vi "ImageThreshold.vi"(2 "Noise standard deviation":dbl format="%.2f", 4 "Sky Scan":dbl[][](graph)=[[180.0, 184.0, 210.0, 205.0, 212.0, 190.0, 183.0, 167.0, 174.0, 172.0, 167.0], [160.0, 192.0, 193.0, 215.0, 200.0, 218.0, 195.0, 180.0, 189.0, 182.0, 179.0], [178.0, 191.0, 222.0, 308.0, 243.0, 199.0, 189.0, 200.0, 192.0, 188.0, 190.0], [170.0, 237.0, 250.0, 257.0, 352.0, 202.0, 187.0, 190.0, 176.0, 182.0, 185.0], [169.0, 264.0, 386.0, 656.0, 212.0, 209.0, 194.0, 190.0, 159.0, 169.0, 190.0], [176.0, 268.0, 1507.0, 3786.0, 748.0, 194.0, 190.0, 209.0, 181.0, 181.0, 174.0], [185.0, 271.0, 1969.0, 5368.0, 1397.0, 218.0, 210.0, 173.0, 194.0, 182.0, 194.0], [185.0, 236.0, 1172.0, 3209.0, 836.0, 187.0, 207.0, 185.0, 179.0, 191.0, 192.0], [169.0, 235.0, 428.0, 829.0, 280.0, 204.0, 175.0, 179.0, 169.0, 195.0, 199.0], [181.0, 195.0, 248.0, 349.0, 318.0, 185.0, 187.0, 188.0, 183.0, 184.0, 197.0], [170.0, 181.0, 186.0, 230.0, 225.0, 199.0, 191.0, 174.0, 181.0, 178.0, 184.0]]) -> (0 "Something ?":bool, 1 "Sky map threshold":dbl[][](graph)=[[180.0, 184.0, 210.0, 205.0, 212.0, 190.0, 183.0, 167.0, 174.0, 172.0, 167.0], [160.0, 192.0, 193.0, 215.0, 200.0, 218.0, 195.0, 180.0, 189.0, 182.0, 179.0], [178.0, 191.0, 222.0, 308.0, 243.0, 199.0, 189.0, 200.0, 192.0, 188.0, 190.0], [170.0, 237.0, 250.0, 257.0, 352.0, 202.0, 187.0, 190.0, 176.0, 182.0, 185.0], [169.0, 264.0, 386.0, 656.0, 212.0, 209.0, 194.0, 190.0, 159.0, 169.0, 190.0], [176.0, 268.0, 1507.0, 3786.0, 748.0, 194.0, 190.0, 209.0, 181.0, 181.0, 174.0], [185.0, 271.0, 1969.0, 5368.0, 1397.0, 218.0, 210.0, 173.0, 194.0, 182.0, 194.0], [185.0, 236.0, 1172.0, 3209.0, 836.0, 187.0, 207.0, 185.0, 179.0, 191.0, 192.0], [169.0, 235.0, 428.0, 829.0, 280.0, 204.0, 175.0, 179.0, 169.0, 195.0, 199.0], [181.0, 195.0, 248.0, 349.0, 318.0, 185.0, 187.0, 188.0, 183.0, 184.0, 197.0], [170.0, 181.0, 186.0, 230.0, 225.0, 199.0, 191.0, 174.0, 181.0, 178.0, 184.0]])   [LabVIEW 2009]
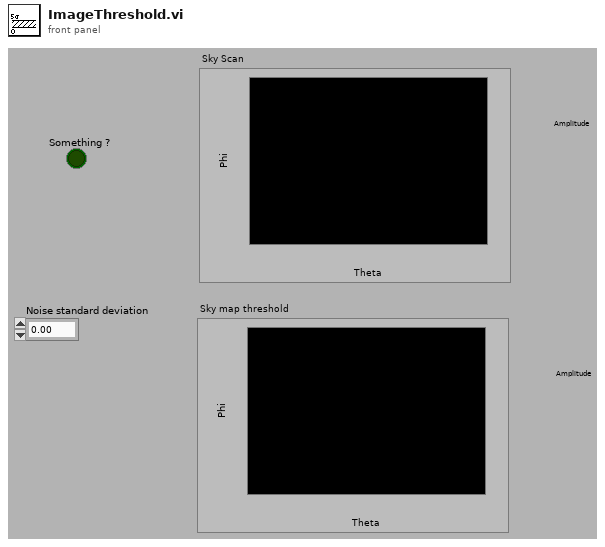
[diagram p1: front panel]
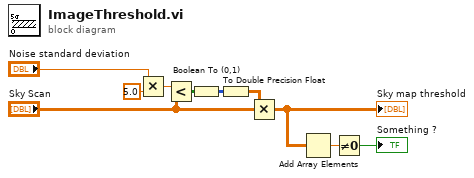
[diagram p0: block diagram]
diagram:
  n1 = Multiply(x="Noise standard deviation", y=5.0) -> (x*y=w7:dbl)
  n2 = Less?(x=w7, y="Sky Scan") -> (x < y?=w9:bool[][])
  n3 = Boolean To (0,1)(Boolean=w9) -> (0, 1=w10:i16[][])
  n4 = To Double Precision Float(number=w10) -> (double precision float=w3:dbl[][])
  n5 = Multiply(x=w3, y="Sky Scan") -> (x*y=w5:dbl[][])
  "Sky map threshold" <- w5
  n6 = Add Array Elements(numeric array=w5) -> (sum=w4:dbl)
  n7 = Not Equal To 0?(x=w4) -> (x != 0?=→"Something ?":bool)
